vi "Climb_Motors.vi"(4 "Driver - Right Thumb":bool, 6 "Driver - Left Thumb":bool, 8 "Driver - Trigger":bool, 9 "Driver - Left Top left":bool, 10 "Driver - Right Top Right":bool, 11 "Driver - Right Top Left":bool) -> ()   [LabVIEW 2020]
uses:
  <vilib>/Rock Robotics/WPI/ThirdParty/Phoenix-LabVIEW/Motor Controller/Controls/CTRE_Phoenix_MotorControl_ControlMode.ctl
  <vilib>/Rock Robotics/Network Tables/NT Read String.vi
panel:
  in  "Low 4":dbl=150000.0
  in  "Low 3":dbl=150000.0
  in  "High 4":dbl
  in  "High 3":dbl
  in  "Traversal 2":dbl
  in  "Traversal 1":dbl
  in  "High 2":dbl
  in  "High 1":dbl
  in  "Mid 2":dbl=400000.0
  in  "Mid 1":dbl=400000.0
  in  "Low 2":dbl=150000.0
  in  "Low 1":dbl=150000.0
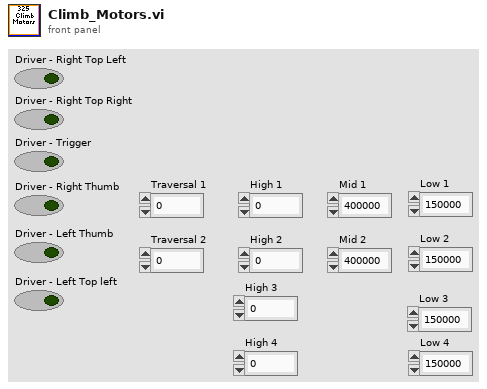
[diagram p1: front panel]
types:
  T1 = typedef "WPI_MotorControlDeviceRef.ctl" = cluster{"DeviceStatus":errorcluster, "Type":T2, "PWM":cluster{"PWM Channel":T3, "DeadBand":T4}, "CAN":cluster{"Device Number":u8, "SetOutput VI Ref":variant, "GetOutput VI Ref":variant, "Enable VI Ref":variant, "Disable VI Ref":variant, "Data":variant}, "Invert":bool, "DIO PWM":cluster{"PWM \"Enable\" Channel":T3, "DIOChannel":T5, "PWM Rate":dbl}}
  T2 = typedef "WPI_MotorControlType.ctl" = enum16{"PWM", "CAN", "DIO PWM"}
  T3 = typedef "FPGA_DIOPWMChannel.ctl" = enum8{"PWM 0", "PWM 1", "PWM 2", "PWM 3", "PWM 4", "PWM 5", "PWM 6", "PWM 7", "PWM 8", "PWM 9", "PWM MXP 0", "PWM MXP 1", "PWM MXP 2", "PWM MXP 3", "PWM MXP 4", "PWM MXP 5", "PWM MXP 6", "PWM MXP 7", "PWM MXP 8", "PWM MXP 9", "Invalid"}
  T4 = typedef "WPI_PWMDeadband.ctl" = cluster{"Name":string, "maxPositivePwm":i32, "minPositivePwm":i32, "centerPwm":i32, "maxNegativePwm":i32, "minNegativePwm":i32, "angularRange":u16}
  T5 = typedef "FPGA_DIOChannel.ctl" = enum8{"DIO 0", "DIO 1", "DIO 2", "DIO 3", "DIO 4", "DIO 5", "DIO 6", "DIO 7", "DIO 8", "DIO 9", "DIO MXP 0", "DIO MXP 1", "DIO MXP 2", "DIO MXP 3", "DIO MXP 4", "DIO MXP 5", "DIO MXP 6", "DIO MXP 7", "DIO MXP 8", "DIO MXP 9", "DIO MXP 10", "DIO MXP 11", "DIO MXP 12", "DIO MXP 13", "DIO MXP 14", "DIO MXP 15", "SPI Port CS1", "SPI Port CS2", "SPI Port CS3", "SPI Port MISO", "SPI Port MOSI", "Invalid"}
  T6 = typedef "CTRE_Phoenix_MotorControl_ControlMode.ctl" = u16
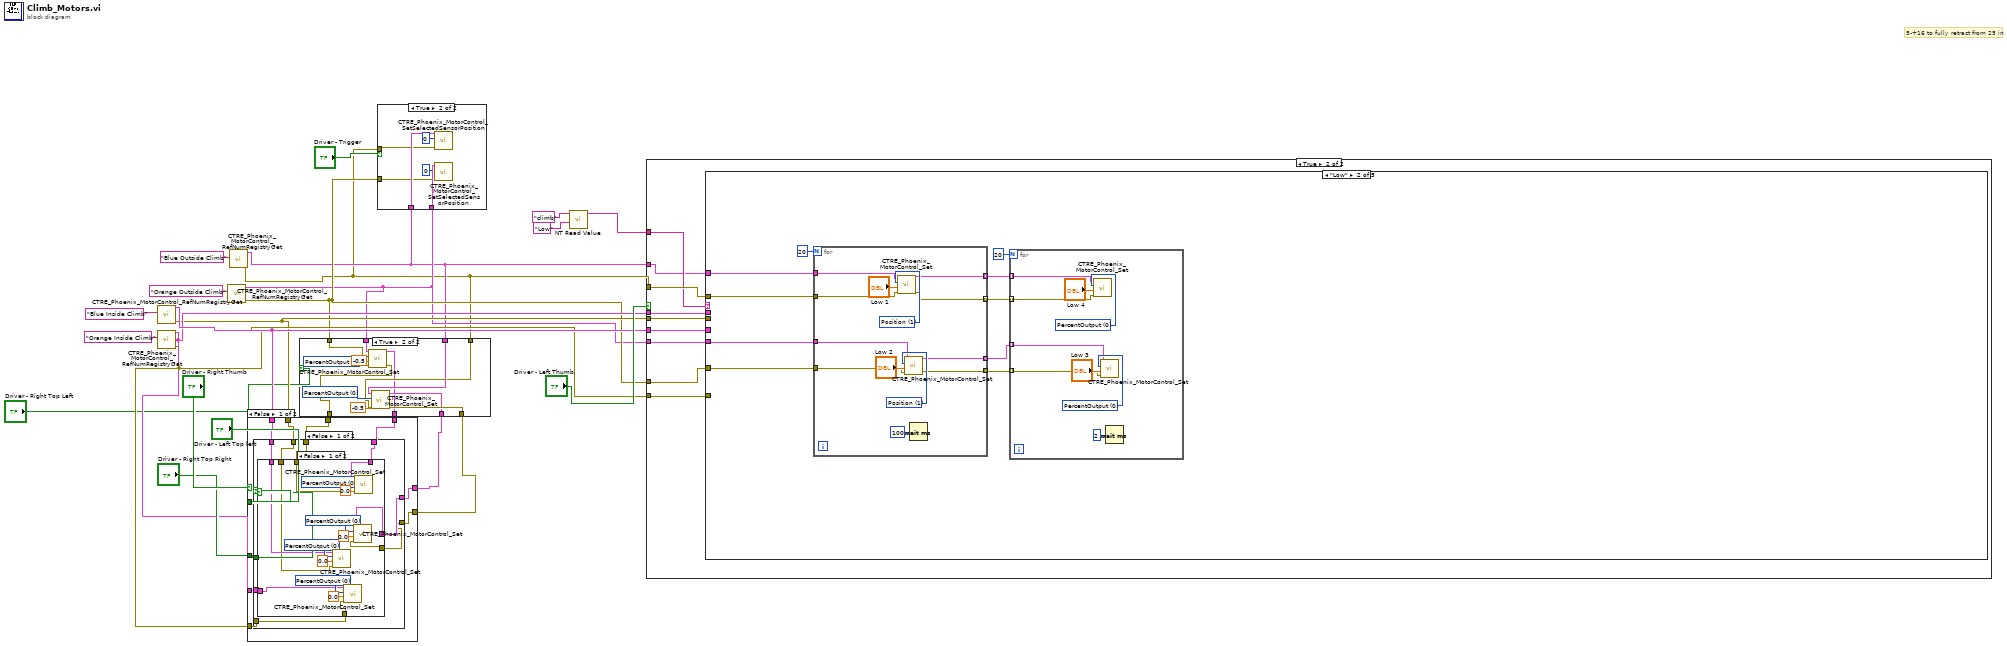
[diagram p0: block diagram]
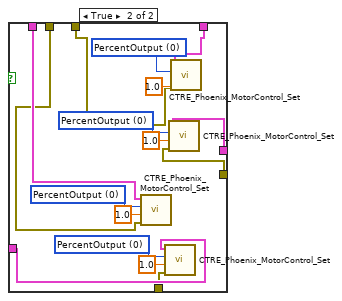
[diagram p3: hidden frame]
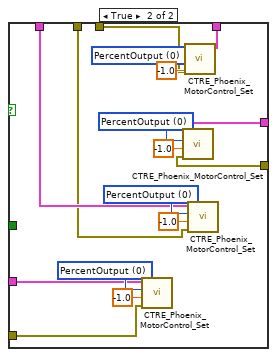
[diagram p4: hidden frame]
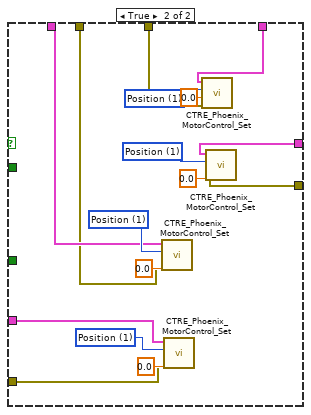
[diagram p5: hidden frame]
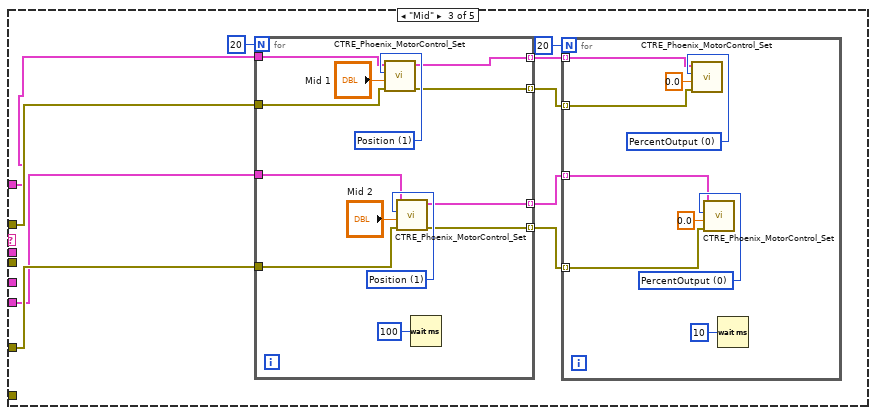
[diagram p8: hidden frame]
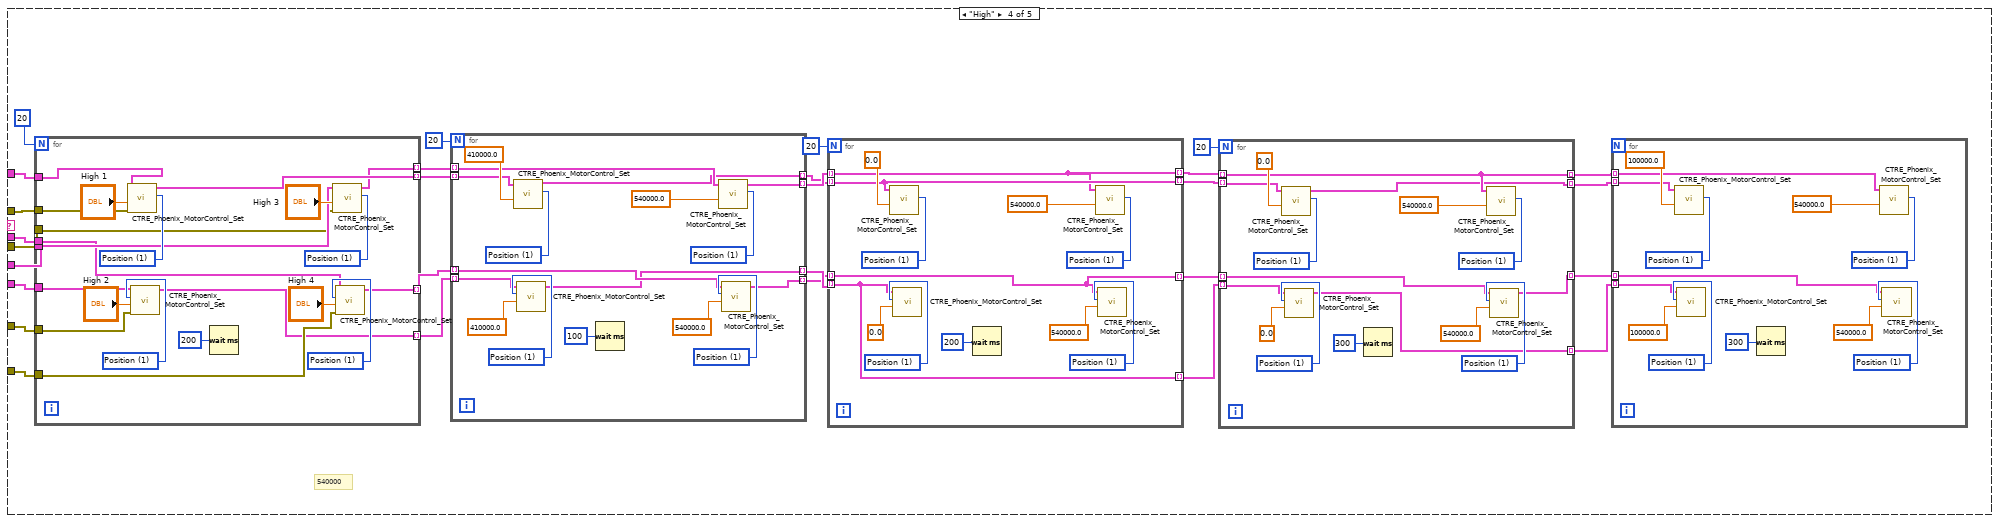
[diagram p9: hidden frame]
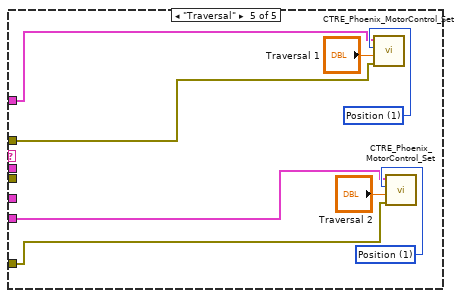
[diagram p10: hidden frame]
diagram:
  # "5-+16 to fully retract from 25 in"
  n1 = call <vilib>:"CTRE_Phoenix_MotorControl_RefNumRegistryGet.vi"("refnum name"="Orange Inside Climb") -> ("error out"=w11:errorcluster, "PhoenixMotorControlDevRef"=w12:T1)  [unwired: 9 in]
  n2 = call <vilib>:"CTRE_Phoenix_MotorControl_RefNumRegistryGet.vi"("refnum name"="Blue Inside Climb") -> ("error out"=w10:errorcluster, "PhoenixMotorControlDevRef"=w13:T1)  [unwired: 9 in]
  n3 = call <vilib>:"CTRE_Phoenix_MotorControl_RefNumRegistryGet.vi"("refnum name"="Orange Outside Climb") -> ("error out"=w9:errorcluster, "PhoenixMotorControlDevRef"=w7:T1)  [unwired: 9 in]
  n4 = call <vilib>:"CTRE_Phoenix_MotorControl_RefNumRegistryGet.vi"("refnum name"="Blue Outside Climb") -> ("error out"=w2:errorcluster, "PhoenixMotorControlDevRef"=w4:T1)  [unwired: 9 in]
  n5 = case shown="True" "Driver - Right Top Left" {
    tunnel: w9 -> [w29 w36]
    tunnel: [w29 w30] -> w8
    tunnel: w7 -> [w28 w37]
    tunnel: [w28 w31] -> w6
    tunnel: [w27 w32] -> w5
    tunnel: w4 -> [w27 w35]
    tunnel: [w26 w33] -> w3
    tunnel: w2 -> [w26 w34]
    frame False {
    }
    frame True {
      w40 = T6 0 items=["PercentOutput"=0, "Position"=1, "Velocity"=2, "Current"=3, "Follower"=5, "MotionProfile"=6, "MotionMagic"=7, "MotionProfileArc"=10, "Disabled"=15] ("Control Mode")
      w41 = T6 0 items=["PercentOutput"=0, "Position"=1, "Velocity"=2, "Current"=3, "Follower"=5, "MotionProfile"=6, "MotionMagic"=7, "MotionProfileArc"=10, "Disabled"=15] ("Control Mode")
      n6 = call <vilib>:"CTRE_Phoenix_MotorControl_Set.vi"("error in (no error)"=w36, "Output"=-0.5, "Control Mode"=w40, "PhoenixMotorControlDevRef"=w37) -> ("error out"=w30:errorcluster, "PhoenixMotorControlDevRef"=w31:T1)  [unwired: 6 in]
      n7 = call <vilib>:"CTRE_Phoenix_MotorControl_Set.vi"("error in (no error)"=w34, "Output"=-0.5, "Control Mode"=w41, "PhoenixMotorControlDevRef"=w35) -> ("error out"=w33:errorcluster, "PhoenixMotorControlDevRef"=w32:T1)  [unwired: 6 in]
    }
  }
  n8 = case shown="False" "Driver - Right Thumb" {
    tunnel: w6 -> [w50 w120]
    tunnel: w8 -> [w49 w119]
    tunnel: w5 -> [w48 w118]
    tunnel: w3 -> [w47 w117]
    tunnel: "Driver - Left Top left" -> [w51 _]
    tunnel: "Driver - Right Top Right" -> [w46 _]
    tunnel: w13 -> [w45 w114]
    tunnel: w10 -> [w44 w113]
    tunnel: w12 -> [w43 w110]
    tunnel: w11 -> [w42 w109]
    frame False {
      n9 = case shown="False" w51 {
        tunnel: w50 -> [w59 w104]
        tunnel: w49 -> [w58 w103]
        tunnel: w48 -> [w57 w102]
        tunnel: w47 -> [w56 w101]
        tunnel: w46 -> [w60 _]
        tunnel: w45 -> [w55 w98]
        tunnel: w44 -> [w54 w97]
        tunnel: w43 -> [w53 w94]
        tunnel: w42 -> [w52 w93]
        frame False {
          n10 = case shown="False" w60 {
            tunnel: w59 -> [w72 w85]
            tunnel: w58 -> [w71 w86]
            tunnel: w57 -> [w70 w87]
            tunnel: w56 -> [w69 w88]
            tunnel: w55 -> [w66 w82]
            tunnel: w54 -> [w65 w81]
            tunnel: w53 -> [w62 w78]
            tunnel: w52 -> [w61 w77]
            frame False {
              w64 = T6 0 items=["PercentOutput"=0, "Position"=1, "Velocity"=2, "Current"=3, "Follower"=5, "MotionProfile"=6, "MotionMagic"=7, "MotionProfileArc"=10, "Disabled"=15] ("Control Mode")
              w68 = T6 0 items=["PercentOutput"=0, "Position"=1, "Velocity"=2, "Current"=3, "Follower"=5, "MotionProfile"=6, "MotionMagic"=7, "MotionProfileArc"=10, "Disabled"=15] ("Control Mode")
              w75 = T6 0 items=["PercentOutput"=0, "Position"=1, "Velocity"=2, "Current"=3, "Follower"=5, "MotionProfile"=6, "MotionMagic"=7, "MotionProfileArc"=10, "Disabled"=15] ("Control Mode")
              w76 = T6 0 items=["PercentOutput"=0, "Position"=1, "Velocity"=2, "Current"=3, "Follower"=5, "MotionProfile"=6, "MotionMagic"=7, "MotionProfileArc"=10, "Disabled"=15] ("Control Mode")
              n11 = call <vilib>:"CTRE_Phoenix_MotorControl_Set.vi"("error in (no error)"=w65, "Output"=0.0, "Control Mode"=w68, "PhoenixMotorControlDevRef"=w66) -> ()  [unwired: 6 in, 2 out]
              n12 = call <vilib>:"CTRE_Phoenix_MotorControl_Set.vi"("error in (no error)"=w61, "Output"=0.0, "Control Mode"=w64, "PhoenixMotorControlDevRef"=w62) -> ()  [unwired: 6 in, 2 out]
              n13 = call <vilib>:"CTRE_Phoenix_MotorControl_Set.vi"("error in (no error)"=w69, "Output"=0.0, "Control Mode"=w76, "PhoenixMotorControlDevRef"=w70) -> ()  [unwired: 6 in, 2 out]
              n14 = call <vilib>:"CTRE_Phoenix_MotorControl_Set.vi"("error in (no error)"=w71, "Output"=0.0, "Control Mode"=w75, "PhoenixMotorControlDevRef"=w72) -> ()  [unwired: 6 in, 2 out]
            }
            frame True {
              w80 = T6 0 items=["PercentOutput"=0, "Position"=1, "Velocity"=2, "Current"=3, "Follower"=5, "MotionProfile"=6, "MotionMagic"=7, "MotionProfileArc"=10, "Disabled"=15] ("Control Mode")
              w84 = T6 0 items=["PercentOutput"=0, "Position"=1, "Velocity"=2, "Current"=3, "Follower"=5, "MotionProfile"=6, "MotionMagic"=7, "MotionProfileArc"=10, "Disabled"=15] ("Control Mode")
              w91 = T6 0 items=["PercentOutput"=0, "Position"=1, "Velocity"=2, "Current"=3, "Follower"=5, "MotionProfile"=6, "MotionMagic"=7, "MotionProfileArc"=10, "Disabled"=15] ("Control Mode")
              w92 = T6 0 items=["PercentOutput"=0, "Position"=1, "Velocity"=2, "Current"=3, "Follower"=5, "MotionProfile"=6, "MotionMagic"=7, "MotionProfileArc"=10, "Disabled"=15] ("Control Mode")
              n15 = call <vilib>:"CTRE_Phoenix_MotorControl_Set.vi"("error in (no error)"=w81, "Output"=1.0, "Control Mode"=w84, "PhoenixMotorControlDevRef"=w82) -> ()  [unwired: 6 in, 2 out]
              n16 = call <vilib>:"CTRE_Phoenix_MotorControl_Set.vi"("error in (no error)"=w77, "Output"=1.0, "Control Mode"=w80, "PhoenixMotorControlDevRef"=w78) -> ()  [unwired: 6 in, 2 out]
              n17 = call <vilib>:"CTRE_Phoenix_MotorControl_Set.vi"("error in (no error)"=w88, "Output"=1.0, "Control Mode"=w92, "PhoenixMotorControlDevRef"=w87) -> ()  [unwired: 6 in, 2 out]
              n18 = call <vilib>:"CTRE_Phoenix_MotorControl_Set.vi"("error in (no error)"=w86, "Output"=1.0, "Control Mode"=w91, "PhoenixMotorControlDevRef"=w85) -> ()  [unwired: 6 in, 2 out]
            }
          }
        }
        frame True {
          w96 = T6 0 items=["PercentOutput"=0, "Position"=1, "Velocity"=2, "Current"=3, "Follower"=5, "MotionProfile"=6, "MotionMagic"=7, "MotionProfileArc"=10, "Disabled"=15] ("Control Mode")
          w100 = T6 0 items=["PercentOutput"=0, "Position"=1, "Velocity"=2, "Current"=3, "Follower"=5, "MotionProfile"=6, "MotionMagic"=7, "MotionProfileArc"=10, "Disabled"=15] ("Control Mode")
          w107 = T6 0 items=["PercentOutput"=0, "Position"=1, "Velocity"=2, "Current"=3, "Follower"=5, "MotionProfile"=6, "MotionMagic"=7, "MotionProfileArc"=10, "Disabled"=15] ("Control Mode")
          w108 = T6 0 items=["PercentOutput"=0, "Position"=1, "Velocity"=2, "Current"=3, "Follower"=5, "MotionProfile"=6, "MotionMagic"=7, "MotionProfileArc"=10, "Disabled"=15] ("Control Mode")
          n19 = call <vilib>:"CTRE_Phoenix_MotorControl_Set.vi"("error in (no error)"=w93, "Output"=-1.0, "Control Mode"=w96, "PhoenixMotorControlDevRef"=w94) -> ()  [unwired: 6 in, 2 out]
          n20 = call <vilib>:"CTRE_Phoenix_MotorControl_Set.vi"("error in (no error)"=w101, "Output"=-1.0, "Control Mode"=w108, "PhoenixMotorControlDevRef"=w102) -> ()  [unwired: 6 in, 2 out]
          n21 = call <vilib>:"CTRE_Phoenix_MotorControl_Set.vi"("error in (no error)"=w103, "Output"=-1.0, "Control Mode"=w107, "PhoenixMotorControlDevRef"=w104) -> ()  [unwired: 6 in, 2 out]
          n22 = call <vilib>:"CTRE_Phoenix_MotorControl_Set.vi"("error in (no error)"=w97, "Output"=-1.0, "Control Mode"=w100, "PhoenixMotorControlDevRef"=w98) -> ()  [unwired: 6 in, 2 out]
        }
      }
    }
    frame True {
      w111 = T6 1 items=["PercentOutput"=0, "Position"=1, "Velocity"=2, "Current"=3, "Follower"=5, "MotionProfile"=6, "MotionMagic"=7, "MotionProfileArc"=10, "Disabled"=15] ("Control Mode")
      w116 = T6 1 items=["PercentOutput"=0, "Position"=1, "Velocity"=2, "Current"=3, "Follower"=5, "MotionProfile"=6, "MotionMagic"=7, "MotionProfileArc"=10, "Disabled"=15] ("Control Mode")
      w123 = T6 1 items=["PercentOutput"=0, "Position"=1, "Velocity"=2, "Current"=3, "Follower"=5, "MotionProfile"=6, "MotionMagic"=7, "MotionProfileArc"=10, "Disabled"=15] ("Control Mode")
      w124 = T6 1 items=["PercentOutput"=0, "Position"=1, "Velocity"=2, "Current"=3, "Follower"=5, "MotionProfile"=6, "MotionMagic"=7, "MotionProfileArc"=10, "Disabled"=15] ("Control Mode")
      n23 = call <vilib>:"CTRE_Phoenix_MotorControl_Set.vi"("error in (no error)"=w113, "Output"=0.0, "Control Mode"=w116, "PhoenixMotorControlDevRef"=w114) -> ()  [unwired: 6 in, 2 out]
      n24 = call <vilib>:"CTRE_Phoenix_MotorControl_Set.vi"("error in (no error)"=w109, "Output"=0.0, "Control Mode"=w111, "PhoenixMotorControlDevRef"=w110) -> ()  [unwired: 6 in, 2 out]
      n25 = call <vilib>:"CTRE_Phoenix_MotorControl_Set.vi"("error in (no error)"=w119, "Output"=0.0, "Control Mode"=w123, "PhoenixMotorControlDevRef"=w120) -> ()  [unwired: 6 in, 2 out]
      n26 = call <vilib>:"CTRE_Phoenix_MotorControl_Set.vi"("error in (no error)"=w117, "Output"=0.0, "Control Mode"=w124, "PhoenixMotorControlDevRef"=w118) -> ()  [unwired: 6 in, 2 out]
    }
  }
  n27 = case shown="True" "Driver - Trigger" {
    tunnel: w4 -> [_ w130]
    tunnel: w2 -> [_ w129]
    tunnel: w7 -> [_ w128]
    tunnel: w9 -> [_ w127]
    frame False {
    }
    frame True {
      n28 = call <vilib>:"CTRE_Phoenix_MotorControl_SetSelectedSensorPosition.vi"("error in (no error)"=w129, "New Sensor Position"=0, "PhoenixMotorControlDevRef"=w130) -> ()  [unwired: 7 in, 2 out]
      n29 = call <vilib>:"CTRE_Phoenix_MotorControl_SetSelectedSensorPosition.vi"("error in (no error)"=w127, "New Sensor Position"=0, "PhoenixMotorControlDevRef"=w128) -> ()  [unwired: 7 in, 2 out]
    }
  }
  n30 = call-poly <vilib>:"NT Read Value.vi"("Default Value"="Low", "Name"="climb") -> ("String"=w18:string)  [unwired: 8 in, 1 out]
  n31 = case shown="True" "Driver - Left Thumb" {
    tunnel: w4 -> [_ w135]
    tunnel: w2 -> [_ w139]
    tunnel: w7 -> [_ w138]
    tunnel: w9 -> [_ w137]
    tunnel: w18 -> [_ w136]
    tunnel: w13 -> [_ w134]
    tunnel: w12 -> [_ w133]
    tunnel: w11 -> [_ w132]
    tunnel: w10 -> [_ w131]
    frame False {
    }
    frame True {
      n32 = case shown="\"Low\"" w136 {
        tunnel: w139 -> [_ w149 w181 w231 w315]
        tunnel: w138 -> [_ w148 w179 w230 w314]
        tunnel: w137 -> [_ w147 w180 w229 w313]
        tunnel: w135 -> [_ w146 w178 w228 w312]
        tunnel: w134 -> [_ _ _ w227 _]
        tunnel: w133 -> [_ _ _ w226 _]
        tunnel: w132 -> [_ _ _ w225 _]
        tunnel: w131 -> [_ _ _ w224 _]
        frame Default {
        }
        frame "Low" {
          n33 = for {
            N: 20 -> [_]
            tunnel: w149 -> [w169]
            tunnel: w148 -> [w166]
            tunnel: w147 -> [w165]
            tunnel: w146 -> [w164]
            tunnel: [w162] -> w144 mode=indexing
            tunnel: [w161] -> w143 mode=indexing
            tunnel: [w160] -> w142 mode=indexing
            tunnel: [w159] -> w141 mode=indexing
            w167 = T6 1 items=["PercentOutput"=0, "Position"=1, "Velocity"=2, "Current"=3, "Follower"=5, "MotionProfile"=6, "MotionMagic"=7, "MotionProfileArc"=10, "Disabled"=15] ("Control Mode")
            w170 = T6 1 items=["PercentOutput"=0, "Position"=1, "Velocity"=2, "Current"=3, "Follower"=5, "MotionProfile"=6, "MotionMagic"=7, "MotionProfileArc"=10, "Disabled"=15] ("Control Mode")
            n34 = call <vilib>:"CTRE_Phoenix_MotorControl_Set.vi"("error in (no error)"=w169, "Output"="Low 1", "Control Mode"=w170, "PhoenixMotorControlDevRef"=w164) -> ("error out"=w161:errorcluster, "PhoenixMotorControlDevRef"=w162:T1)  [unwired: 6 in]
            n35 = call <vilib>:"CTRE_Phoenix_MotorControl_Set.vi"("error in (no error)"=w165, "Output"="Low 2", "Control Mode"=w167, "PhoenixMotorControlDevRef"=w166) -> ("error out"=w159:errorcluster, "PhoenixMotorControlDevRef"=w160:T1)  [unwired: 6 in]
            n36 = Wait (ms)(milliseconds to wait=u32 100) -> ()  [unwired: 1 out]
          }
          n37 = for {
            N: 20 -> [_]
            tunnel: w143 -> [w156] mode=indexing
            tunnel: w142 -> [w153] mode=indexing
            tunnel: w141 -> [w152] mode=indexing
            tunnel: w144 -> [w151] mode=indexing
            w154 = T6 0 items=["PercentOutput"=0, "Position"=1, "Velocity"=2, "Current"=3, "Follower"=5, "MotionProfile"=6, "MotionMagic"=7, "MotionProfileArc"=10, "Disabled"=15] ("Control Mode")
            w157 = T6 0 items=["PercentOutput"=0, "Position"=1, "Velocity"=2, "Current"=3, "Follower"=5, "MotionProfile"=6, "MotionMagic"=7, "MotionProfileArc"=10, "Disabled"=15] ("Control Mode")
            n38 = call <vilib>:"CTRE_Phoenix_MotorControl_Set.vi"("error in (no error)"=w156, "Output"="Low 4", "Control Mode"=w157, "PhoenixMotorControlDevRef"=w151) -> ()  [unwired: 6 in, 2 out]
            n39 = call <vilib>:"CTRE_Phoenix_MotorControl_Set.vi"("error in (no error)"=w152, "Output"="Low 3", "Control Mode"=w154, "PhoenixMotorControlDevRef"=w153) -> ()  [unwired: 6 in, 2 out]
            n40 = Wait (ms)(milliseconds to wait=u32 2) -> ()  [unwired: 1 out]
          }
        }
        frame "Mid" {
          n41 = for {
            N: 20 -> [_]
            tunnel: w181 -> [w199]
            tunnel: w180 -> [w198]
            tunnel: w179 -> [w197]
            tunnel: w178 -> [w196]
            tunnel: [w194] -> w176 mode=indexing
            tunnel: [w193] -> w175 mode=indexing
            tunnel: [w192] -> w174 mode=indexing
            tunnel: [w191] -> w173 mode=indexing
            w200 = T6 1 items=["PercentOutput"=0, "Position"=1, "Velocity"=2, "Current"=3, "Follower"=5, "MotionProfile"=6, "MotionMagic"=7, "MotionProfileArc"=10, "Disabled"=15] ("Control Mode")
            w202 = T6 1 items=["PercentOutput"=0, "Position"=1, "Velocity"=2, "Current"=3, "Follower"=5, "MotionProfile"=6, "MotionMagic"=7, "MotionProfileArc"=10, "Disabled"=15] ("Control Mode")
            n42 = call <vilib>:"CTRE_Phoenix_MotorControl_Set.vi"("error in (no error)"=w199, "Output"="Mid 1", "Control Mode"=w202, "PhoenixMotorControlDevRef"=w196) -> ("error out"=w192:errorcluster, "PhoenixMotorControlDevRef"=w191:T1)  [unwired: 6 in]
            n43 = call <vilib>:"CTRE_Phoenix_MotorControl_Set.vi"("error in (no error)"=w198, "Output"="Mid 2", "Control Mode"=w200, "PhoenixMotorControlDevRef"=w197) -> ("error out"=w194:errorcluster, "PhoenixMotorControlDevRef"=w193:T1)  [unwired: 6 in]
            n44 = Wait (ms)(milliseconds to wait=u32 100) -> ()  [unwired: 1 out]
          }
          n45 = for {
            N: 20 -> [_]
            tunnel: w174 -> [w188] mode=indexing
            tunnel: w176 -> [w187] mode=indexing
            tunnel: w175 -> [w186] mode=indexing
            tunnel: w173 -> [w185] mode=indexing
            w189 = T6 0 items=["PercentOutput"=0, "Position"=1, "Velocity"=2, "Current"=3, "Follower"=5, "MotionProfile"=6, "MotionMagic"=7, "MotionProfileArc"=10, "Disabled"=15] ("Control Mode")
            w190 = T6 0 items=["PercentOutput"=0, "Position"=1, "Velocity"=2, "Current"=3, "Follower"=5, "MotionProfile"=6, "MotionMagic"=7, "MotionProfileArc"=10, "Disabled"=15] ("Control Mode")
            n46 = call <vilib>:"CTRE_Phoenix_MotorControl_Set.vi"("error in (no error)"=w188, "Output"=0.0, "Control Mode"=w190, "PhoenixMotorControlDevRef"=w185) -> ()  [unwired: 6 in, 2 out]
            n47 = call <vilib>:"CTRE_Phoenix_MotorControl_Set.vi"("error in (no error)"=w187, "Output"=0.0, "Control Mode"=w189, "PhoenixMotorControlDevRef"=w186) -> ()  [unwired: 6 in, 2 out]
            n48 = Wait (ms)(milliseconds to wait=u32 10) -> ()  [unwired: 1 out]
          }
        }
        frame "High" {
          # "540000"
          n49 = for {
            N: 20 -> [_]
            tunnel: w231 -> [w307]
            tunnel: w230 -> [w306]
            tunnel: w229 -> [w305]
            tunnel: w228 -> [w295]
            tunnel: w227 -> [w300]
            tunnel: w226 -> [w299]
            tunnel: w225 -> [w298]
            tunnel: w224 -> [w297]
            tunnel: [w294] -> w222 mode=indexing
            tunnel: [w293] -> w221 mode=indexing
            tunnel: [w292] -> w220 mode=indexing
            tunnel: [w291] -> w219 mode=indexing
            w301 = T6 1 items=["PercentOutput"=0, "Position"=1, "Velocity"=2, "Current"=3, "Follower"=5, "MotionProfile"=6, "MotionMagic"=7, "MotionProfileArc"=10, "Disabled"=15] ("Control Mode")
            w303 = T6 1 items=["PercentOutput"=0, "Position"=1, "Velocity"=2, "Current"=3, "Follower"=5, "MotionProfile"=6, "MotionMagic"=7, "MotionProfileArc"=10, "Disabled"=15] ("Control Mode")
            w308 = T6 1 items=["PercentOutput"=0, "Position"=1, "Velocity"=2, "Current"=3, "Follower"=5, "MotionProfile"=6, "MotionMagic"=7, "MotionProfileArc"=10, "Disabled"=15] ("Control Mode")
            w310 = T6 1 items=["PercentOutput"=0, "Position"=1, "Velocity"=2, "Current"=3, "Follower"=5, "MotionProfile"=6, "MotionMagic"=7, "MotionProfileArc"=10, "Disabled"=15] ("Control Mode")
            n50 = call <vilib>:"CTRE_Phoenix_MotorControl_Set.vi"("error in (no error)"=w307, "Output"="High 1", "Control Mode"=w310, "PhoenixMotorControlDevRef"=w295) -> ("PhoenixMotorControlDevRef"=w294:T1)  [unwired: 6 in, 1 out]
            n51 = call <vilib>:"CTRE_Phoenix_MotorControl_Set.vi"("error in (no error)"=w305, "Output"="High 2", "Control Mode"=w308, "PhoenixMotorControlDevRef"=w306) -> ("PhoenixMotorControlDevRef"=w292:T1)  [unwired: 6 in, 1 out]
            n52 = Wait (ms)(milliseconds to wait=u32 200) -> ()  [unwired: 1 out]
            n53 = call <vilib>:"CTRE_Phoenix_MotorControl_Set.vi"("error in (no error)"=w297, "Output"="High 3", "Control Mode"=w303, "PhoenixMotorControlDevRef"=w300) -> ("PhoenixMotorControlDevRef"=w293:T1)  [unwired: 6 in, 1 out]
            n54 = call <vilib>:"CTRE_Phoenix_MotorControl_Set.vi"("error in (no error)"=w298, "Output"="High 4", "Control Mode"=w301, "PhoenixMotorControlDevRef"=w299) -> ("PhoenixMotorControlDevRef"=w291:T1)  [unwired: 6 in, 1 out]
          }
          n55 = for {
            N: 20 -> [_]
            tunnel: w222 -> [w281] mode=indexing
            tunnel: w221 -> [w280] mode=indexing
            tunnel: w220 -> [w279] mode=indexing
            tunnel: w219 -> [w278] mode=indexing
            tunnel: [w277] -> w217 mode=indexing
            tunnel: [w276] -> w216 mode=indexing
            tunnel: [w275] -> w215 mode=indexing
            tunnel: [w274] -> w214 mode=indexing
            w283 = T6 1 items=["PercentOutput"=0, "Position"=1, "Velocity"=2, "Current"=3, "Follower"=5, "MotionProfile"=6, "MotionMagic"=7, "MotionProfileArc"=10, "Disabled"=15] ("Control Mode")
            w285 = T6 1 items=["PercentOutput"=0, "Position"=1, "Velocity"=2, "Current"=3, "Follower"=5, "MotionProfile"=6, "MotionMagic"=7, "MotionProfileArc"=10, "Disabled"=15] ("Control Mode")
            w287 = T6 1 items=["PercentOutput"=0, "Position"=1, "Velocity"=2, "Current"=3, "Follower"=5, "MotionProfile"=6, "MotionMagic"=7, "MotionProfileArc"=10, "Disabled"=15] ("Control Mode")
            w289 = T6 1 items=["PercentOutput"=0, "Position"=1, "Velocity"=2, "Current"=3, "Follower"=5, "MotionProfile"=6, "MotionMagic"=7, "MotionProfileArc"=10, "Disabled"=15] ("Control Mode")
            n56 = call <vilib>:"CTRE_Phoenix_MotorControl_Set.vi"("Output"=410000.0 ("High 8"), "Control Mode"=w289, "PhoenixMotorControlDevRef"=w281) -> ("PhoenixMotorControlDevRef"=w276:T1)  [unwired: 7 in, 1 out]
            n57 = call <vilib>:"CTRE_Phoenix_MotorControl_Set.vi"("Output"=410000.0 ("High 7"), "Control Mode"=w287, "PhoenixMotorControlDevRef"=w279) -> ("PhoenixMotorControlDevRef"=w275:T1)  [unwired: 7 in, 1 out]
            n58 = Wait (ms)(milliseconds to wait=u32 100) -> ()  [unwired: 1 out]
            n59 = call <vilib>:"CTRE_Phoenix_MotorControl_Set.vi"("Output"=540000.0 ("High 6"), "Control Mode"=w285, "PhoenixMotorControlDevRef"=w280) -> ("PhoenixMotorControlDevRef"=w277:T1)  [unwired: 7 in, 1 out]
            n60 = call <vilib>:"CTRE_Phoenix_MotorControl_Set.vi"("Output"=540000.0 ("High 5"), "Control Mode"=w283, "PhoenixMotorControlDevRef"=w278) -> ("PhoenixMotorControlDevRef"=w274:T1)  [unwired: 7 in, 1 out]
          }
          n61 = for {
            N: 20 -> [_]
            tunnel: w216 -> [w264] mode=indexing
            tunnel: w217 -> [w263] mode=indexing
            tunnel: w215 -> [w261] mode=indexing
            tunnel: w214 -> [w262] mode=indexing
            tunnel: [w264] -> w211 mode=indexing
            tunnel: [w263] -> w210 mode=indexing
            tunnel: [w262] -> w209 mode=indexing
            tunnel: [w261] -> w208 mode=indexing
            w266 = T6 1 items=["PercentOutput"=0, "Position"=1, "Velocity"=2, "Current"=3, "Follower"=5, "MotionProfile"=6, "MotionMagic"=7, "MotionProfileArc"=10, "Disabled"=15] ("Control Mode")
            w268 = T6 1 items=["PercentOutput"=0, "Position"=1, "Velocity"=2, "Current"=3, "Follower"=5, "MotionProfile"=6, "MotionMagic"=7, "MotionProfileArc"=10, "Disabled"=15] ("Control Mode")
            w270 = T6 1 items=["PercentOutput"=0, "Position"=1, "Velocity"=2, "Current"=3, "Follower"=5, "MotionProfile"=6, "MotionMagic"=7, "MotionProfileArc"=10, "Disabled"=15] ("Control Mode")
            w272 = T6 1 items=["PercentOutput"=0, "Position"=1, "Velocity"=2, "Current"=3, "Follower"=5, "MotionProfile"=6, "MotionMagic"=7, "MotionProfileArc"=10, "Disabled"=15] ("Control Mode")
            n62 = call <vilib>:"CTRE_Phoenix_MotorControl_Set.vi"("Output"=0.0 ("High 8"), "Control Mode"=w272, "PhoenixMotorControlDevRef"=w264) -> ()  [unwired: 7 in, 2 out]
            n63 = call <vilib>:"CTRE_Phoenix_MotorControl_Set.vi"("Output"=0.0 ("High 7"), "Control Mode"=w270, "PhoenixMotorControlDevRef"=w261) -> ()  [unwired: 7 in, 2 out]
            n64 = Wait (ms)(milliseconds to wait=u32 200) -> ()  [unwired: 1 out]
            n65 = call <vilib>:"CTRE_Phoenix_MotorControl_Set.vi"("Output"=540000.0 ("High 6"), "Control Mode"=w268, "PhoenixMotorControlDevRef"=w263) -> ()  [unwired: 7 in, 2 out]
            n66 = call <vilib>:"CTRE_Phoenix_MotorControl_Set.vi"("Output"=540000.0 ("High 5"), "Control Mode"=w266, "PhoenixMotorControlDevRef"=w262) -> ()  [unwired: 7 in, 2 out]
          }
          n67 = for {
            N: 20 -> [_]
            tunnel: w211 -> [w251] mode=indexing
            tunnel: w210 -> [w248] mode=indexing
            tunnel: w208 -> [w250] mode=indexing
            tunnel: w209 -> [w249] mode=indexing
            tunnel: [w248] -> w207 mode=indexing
            tunnel: [w247] -> w206 mode=indexing
            tunnel: [w246] -> w205 mode=indexing
            tunnel: [w245] -> w204 mode=indexing
            w253 = T6 1 items=["PercentOutput"=0, "Position"=1, "Velocity"=2, "Current"=3, "Follower"=5, "MotionProfile"=6, "MotionMagic"=7, "MotionProfileArc"=10, "Disabled"=15] ("Control Mode")
            w255 = T6 1 items=["PercentOutput"=0, "Position"=1, "Velocity"=2, "Current"=3, "Follower"=5, "MotionProfile"=6, "MotionMagic"=7, "MotionProfileArc"=10, "Disabled"=15] ("Control Mode")
            w257 = T6 1 items=["PercentOutput"=0, "Position"=1, "Velocity"=2, "Current"=3, "Follower"=5, "MotionProfile"=6, "MotionMagic"=7, "MotionProfileArc"=10, "Disabled"=15] ("Control Mode")
            w259 = T6 1 items=["PercentOutput"=0, "Position"=1, "Velocity"=2, "Current"=3, "Follower"=5, "MotionProfile"=6, "MotionMagic"=7, "MotionProfileArc"=10, "Disabled"=15] ("Control Mode")
            n68 = call <vilib>:"CTRE_Phoenix_MotorControl_Set.vi"("Output"=0.0 ("High 8"), "Control Mode"=w259, "PhoenixMotorControlDevRef"=w251) -> ("PhoenixMotorControlDevRef"=w247:T1)  [unwired: 7 in, 1 out]
            n69 = call <vilib>:"CTRE_Phoenix_MotorControl_Set.vi"("Output"=0.0 ("High 7"), "Control Mode"=w257, "PhoenixMotorControlDevRef"=w250) -> ("PhoenixMotorControlDevRef"=w245:T1)  [unwired: 7 in, 1 out]
            n70 = Wait (ms)(milliseconds to wait=u32 300) -> ()  [unwired: 1 out]
            n71 = call <vilib>:"CTRE_Phoenix_MotorControl_Set.vi"("Output"=540000.0 ("High 6"), "Control Mode"=w255, "PhoenixMotorControlDevRef"=w248) -> ()  [unwired: 7 in, 2 out]
            n72 = call <vilib>:"CTRE_Phoenix_MotorControl_Set.vi"("Output"=540000.0 ("High 5"), "Control Mode"=w253, "PhoenixMotorControlDevRef"=w249) -> ("PhoenixMotorControlDevRef"=w246:T1)  [unwired: 7 in, 1 out]
          }
          n73 = for {
            tunnel: w206 -> [w235] mode=indexing
            tunnel: w207 -> [w234] mode=indexing
            tunnel: w204 -> [w233] mode=indexing
            tunnel: w205 -> [w232] mode=indexing
            w237 = T6 1 items=["PercentOutput"=0, "Position"=1, "Velocity"=2, "Current"=3, "Follower"=5, "MotionProfile"=6, "MotionMagic"=7, "MotionProfileArc"=10, "Disabled"=15] ("Control Mode")
            w239 = T6 1 items=["PercentOutput"=0, "Position"=1, "Velocity"=2, "Current"=3, "Follower"=5, "MotionProfile"=6, "MotionMagic"=7, "MotionProfileArc"=10, "Disabled"=15] ("Control Mode")
            w241 = T6 1 items=["PercentOutput"=0, "Position"=1, "Velocity"=2, "Current"=3, "Follower"=5, "MotionProfile"=6, "MotionMagic"=7, "MotionProfileArc"=10, "Disabled"=15] ("Control Mode")
            w243 = T6 1 items=["PercentOutput"=0, "Position"=1, "Velocity"=2, "Current"=3, "Follower"=5, "MotionProfile"=6, "MotionMagic"=7, "MotionProfileArc"=10, "Disabled"=15] ("Control Mode")
            n74 = call <vilib>:"CTRE_Phoenix_MotorControl_Set.vi"("Output"=100000.0 ("High 8"), "Control Mode"=w243, "PhoenixMotorControlDevRef"=w235) -> ()  [unwired: 7 in, 2 out]
            n75 = call <vilib>:"CTRE_Phoenix_MotorControl_Set.vi"("Output"=100000.0 ("High 7"), "Control Mode"=w241, "PhoenixMotorControlDevRef"=w233) -> ()  [unwired: 7 in, 2 out]
            n76 = Wait (ms)(milliseconds to wait=u32 300) -> ()  [unwired: 1 out]
            n77 = call <vilib>:"CTRE_Phoenix_MotorControl_Set.vi"("Output"=540000.0 ("High 6"), "Control Mode"=w239, "PhoenixMotorControlDevRef"=w234) -> ()  [unwired: 7 in, 2 out]
            n78 = call <vilib>:"CTRE_Phoenix_MotorControl_Set.vi"("Output"=540000.0 ("High 5"), "Control Mode"=w237, "PhoenixMotorControlDevRef"=w232) -> ()  [unwired: 7 in, 2 out]
          }
        }
        frame "Traversal" {
          w316 = T6 1 items=["PercentOutput"=0, "Position"=1, "Velocity"=2, "Current"=3, "Follower"=5, "MotionProfile"=6, "MotionMagic"=7, "MotionProfileArc"=10, "Disabled"=15] ("Control Mode")
          w318 = T6 1 items=["PercentOutput"=0, "Position"=1, "Velocity"=2, "Current"=3, "Follower"=5, "MotionProfile"=6, "MotionMagic"=7, "MotionProfileArc"=10, "Disabled"=15] ("Control Mode")
          n79 = call <vilib>:"CTRE_Phoenix_MotorControl_Set.vi"("error in (no error)"=w315, "Output"="Traversal 1", "Control Mode"=w318, "PhoenixMotorControlDevRef"=w312) -> ()  [unwired: 6 in, 2 out]
          n80 = call <vilib>:"CTRE_Phoenix_MotorControl_Set.vi"("error in (no error)"=w313, "Output"="Traversal 2", "Control Mode"=w316, "PhoenixMotorControlDevRef"=w314) -> ()  [unwired: 6 in, 2 out]
        }
      }
    }
  }
